vi "Finalize To Settings.vi"(8 "error in (no error)":errorcluster, 11 "UDPlog Transfer Rx Configuration in":refnum<class "UDPlog Transfer Rx Configuration.lvclass">) -> (0 "error out":errorcluster, 2 "settings":cluster{"key":string, "value":string}[](array[cluster]), 3 "UDPlog Transfer Rx Configuration out":refnum<class "UDPlog Transfer Rx Configuration.lvclass">)   [LabVIEW 2023, in "UDPlog.lvlib" / "UDPlog Transfer Rx Configuration.lvclass"]
uses:
  UDPlog Transfer Rx Configuration.lvclass
  UDPlog Transfer Rx Configuration.lvclass/UDPlog Transfer Rx Configuration.ctl
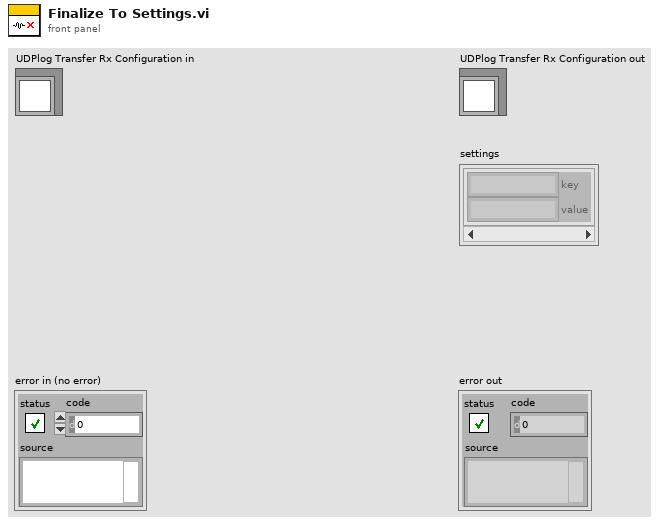
[diagram p1: front panel]
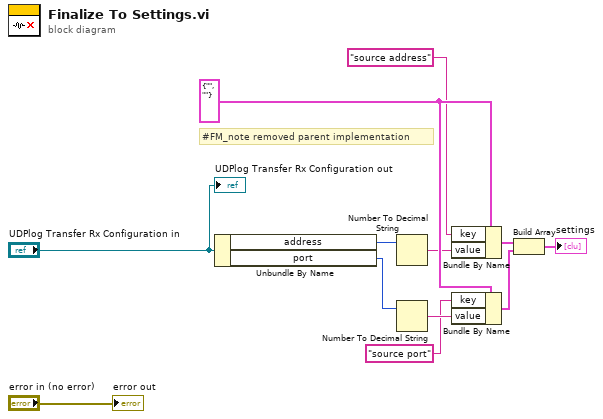
[diagram p0: block diagram]
diagram:
  w11 = cluster{"key":string, "value":string} {"key"="", "value"=""} ("setting")
  # "#FM_note removed parent implementation"
  n1 = Unbundle By Name("UDPlog Transfer Rx Configuration in") -> ("address"=w2:u32, "port"=w1:u16)
  n2 = Number To Decimal String(number=w2) -> (decimal integer string=w5:string)  [unwired: 1 in]
  n3 = Number To Decimal String(number=w1) -> (decimal integer string=w10:string)  [unwired: 1 in]
  n4 = Bundle By Name(cluster=w11, "key"="source address", "value"=w5) -> (w9:cluster{"key":string, "value":string})
  n5 = Bundle By Name(cluster=w11, "key"="source port", "value"=w10) -> (w8:cluster{"key":string, "value":string})
  n6 = Build Array(w9, w8) -> (→"settings":cluster{"key":string, "value":string}[])
  "error out" <- "error in (no error)"
  "UDPlog Transfer Rx Configuration out" <- "UDPlog Transfer Rx Configuration in"
